vi "test_Simulation Recourse Buffer.vi"(8 "error in (no error)":errorcluster) -> (0 "error out":errorcluster, 3 "Passed?":bool)   [LabVIEW 2016]
uses:
  Host/Typedefs/IO Buffer Operation.ctl
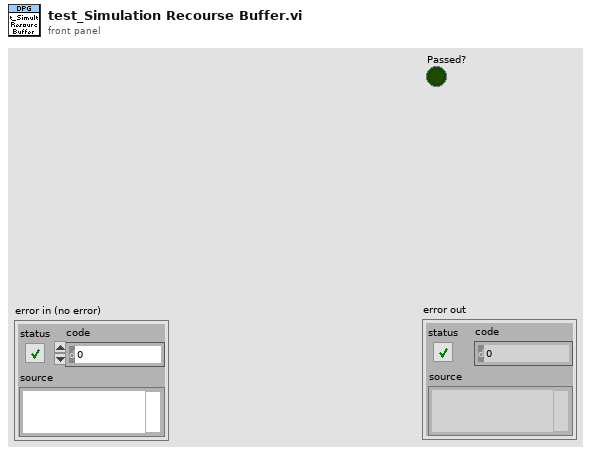
[diagram p1: front panel]
types:
  T1 = typedef "IO Buffer Operation.ctl" = enum16{"Initialize", "Write IO Data_Rd", "Read IO Data_Rd", "Write IO Data_Wr", "Read IO Data_Wr", "Write  IO Data_Dir", "Read  IO Data_Dir", "Write Host to Target FIFO", "Read Host to Target FIFO", "Write Target to Host FIFO", "Read Target to Host FIFO", "Write Monitor Enable?", "Read Monitor Enable?", "Close"}
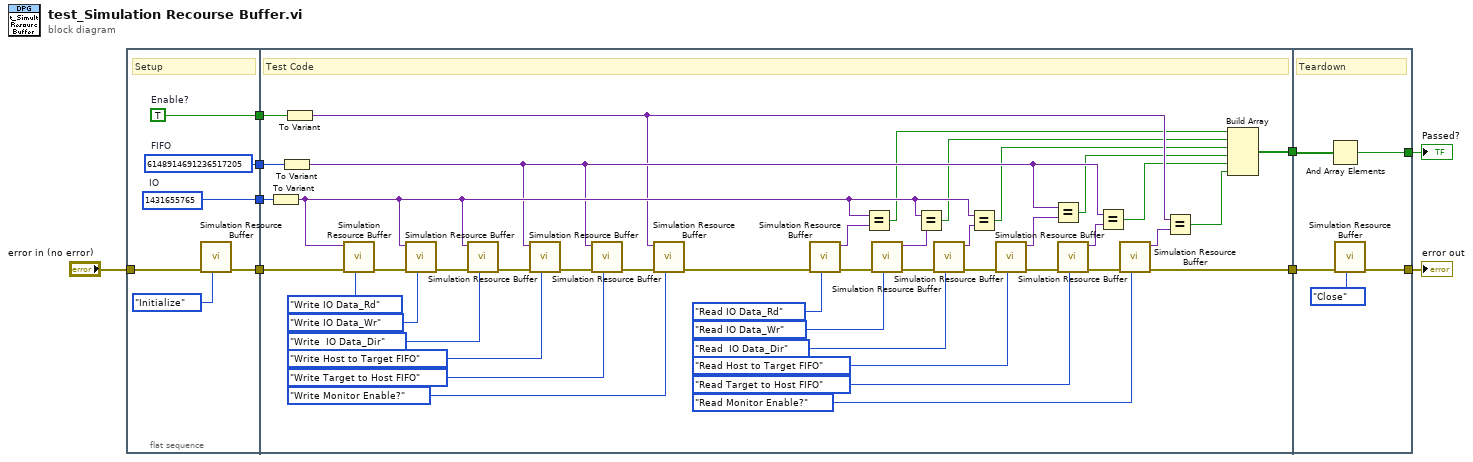
[diagram p0: block diagram]
diagram:
  n1 = flat-sequence {
    tunnel: "error in (no error)" -> [w13]
    tunnel: [w14] -> w9
    tunnel: [w12] -> w5
    tunnel: [w11] -> w4
    tunnel: [w10] -> w3
    tunnel: w9 -> [w59]
    tunnel: [w35] -> w6
    tunnel: w5 -> [w34]
    tunnel: w4 -> [w33]
    tunnel: w3 -> [w32]
    tunnel: [w16] -> w2
    tunnel: [w64] -> w7
    tunnel: w6 -> [w62]
    tunnel: w2 -> [w61]
    tunnel: [w60] -> w1
    frame #0 {
      w10 = TRUE  # Enable?
      w11 = u64 6148914691236517205  # FIFO
      w12 = u32 1431655765  # IO
      # "Setup"
      n2 = call "Simulation Resource Buffer.vi"("IO Buffer Operation"=IO_Buffer_Operation."Initialize", "error in (no error)"=w13) -> ("error out"=w14:errorcluster)  [unwired: 7 in, 2 out]
    }
    frame #1 {
      # "Test Code"
      n3 = To Variant(anything=w34) -> (Variant=w28:variant)
      n4 = To Variant(anything=w33) -> (Variant=w25:variant)
      n5 = To Variant(anything=w32) -> (Variant=w23:variant)
      n6 = call "Simulation Resource Buffer.vi"("IO Buffer Operation"=IO_Buffer_Operation."Write IO Data_Rd", "error in (no error)"=w59, "Data in"=w28) -> ("error out"=w57:errorcluster)  [unwired: 6 in, 2 out]
      n7 = call "Simulation Resource Buffer.vi"("IO Buffer Operation"=IO_Buffer_Operation."Write IO Data_Wr", "error in (no error)"=w57, "Data in"=w28) -> ("error out"=w55:errorcluster)  [unwired: 6 in, 2 out]
      n8 = call "Simulation Resource Buffer.vi"("IO Buffer Operation"=IO_Buffer_Operation."Write  IO Data_Dir", "error in (no error)"=w55, "Data in"=w28) -> ("error out"=w53:errorcluster)  [unwired: 6 in, 2 out]
      n9 = call "Simulation Resource Buffer.vi"("IO Buffer Operation"=IO_Buffer_Operation."Write Host to Target FIFO", "error in (no error)"=w53, "Data in"=w25) -> ("error out"=w51:errorcluster)  [unwired: 6 in, 2 out]
      n10 = call "Simulation Resource Buffer.vi"("IO Buffer Operation"=IO_Buffer_Operation."Write Target to Host FIFO", "error in (no error)"=w51, "Data in"=w25) -> ("error out"=w49:errorcluster)  [unwired: 6 in, 2 out]
      n11 = call "Simulation Resource Buffer.vi"("IO Buffer Operation"=IO_Buffer_Operation."Write Monitor Enable?", "error in (no error)"=w49, "Data in"=w23) -> ("error out"=w36:errorcluster)  [unwired: 6 in, 2 out]
      n12 = call "Simulation Resource Buffer.vi"("IO Buffer Operation"=IO_Buffer_Operation."Read IO Data_Rd", "error in (no error)"=w36) -> ("error out"=w43:errorcluster, "Data out"=w31:variant)  [unwired: 7 in, 1 out]
      n13 = Equal?(x=w28, y=w31) -> (x = y?=w22:bool)
      n14 = call "Simulation Resource Buffer.vi"("IO Buffer Operation"=IO_Buffer_Operation."Read IO Data_Wr", "error in (no error)"=w43) -> ("error out"=w44:errorcluster, "Data out"=w30:variant)  [unwired: 7 in, 1 out]
      n15 = Equal?(x=w28, y=w30) -> (x = y?=w21:bool)
      n16 = call "Simulation Resource Buffer.vi"("IO Buffer Operation"=IO_Buffer_Operation."Read  IO Data_Dir", "error in (no error)"=w44) -> ("error out"=w45:errorcluster, "Data out"=w29:variant)  [unwired: 7 in, 1 out]
      n17 = Equal?(x=w28, y=w29) -> (x = y?=w20:bool)
      n18 = call "Simulation Resource Buffer.vi"("IO Buffer Operation"=IO_Buffer_Operation."Read Host to Target FIFO", "error in (no error)"=w45) -> ("error out"=w46:errorcluster, "Data out"=w27:variant)  [unwired: 7 in, 1 out]
      n19 = Equal?(x=w25, y=w27) -> (x = y?=w19:bool)
      n20 = call "Simulation Resource Buffer.vi"("IO Buffer Operation"=IO_Buffer_Operation."Read Target to Host FIFO", "error in (no error)"=w46) -> ("error out"=w47:errorcluster, "Data out"=w26:variant)  [unwired: 7 in, 1 out]
      n21 = Equal?(x=w25, y=w26) -> (x = y?=w18:bool)
      n22 = call "Simulation Resource Buffer.vi"("IO Buffer Operation"=IO_Buffer_Operation."Read Monitor Enable?", "error in (no error)"=w47) -> ("error out"=w35:errorcluster, "Data out"=w24:variant)  [unwired: 7 in, 1 out]
      n23 = Equal?(x=w23, y=w24) -> (x = y?=w17:bool)
      n24 = Build Array(w22, w21, w20, w19, w18, w17) -> (w16:bool[])
    }
    frame #2 {
      # "Teardown"
      n25 = And Array Elements(Boolean array=w61) -> (logical AND=w60:bool)
      n26 = call "Simulation Resource Buffer.vi"("IO Buffer Operation"=IO_Buffer_Operation."Close", "error in (no error)"=w62) -> ("error out"=w64:errorcluster)  [unwired: 7 in, 2 out]
    }
  }
  "error out" <- w7
  "Passed?" <- w1
